vi "test_sound.vi"() -> ()   [LabVIEW 2019]
panel:
  in  "stop":bool
  out "frequency":dbl
  out "touch":dbl
  in  "stop (F)":bool
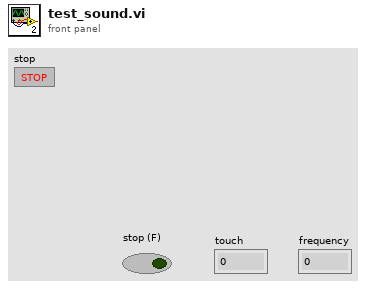
[diagram p1: front panel]
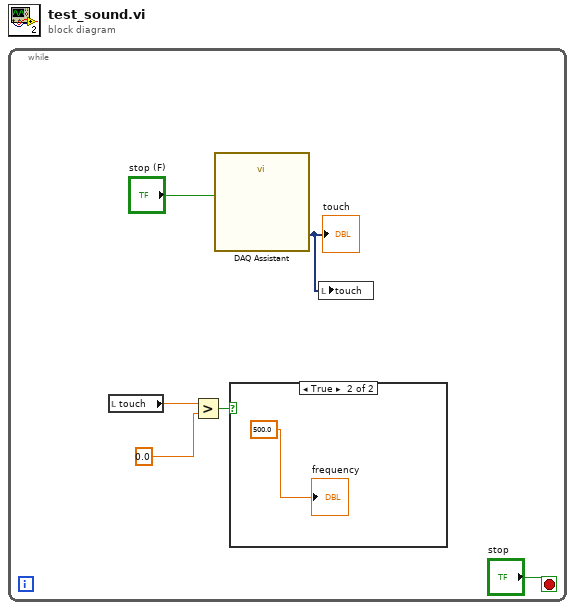
[diagram p0: block diagram]
diagram:
  n1 = while {
    stop <- "stop" stop-if-true
    n2 = local read "touch"() -> (w6:dbl)
    n3 = Greater?(x=w6, y=0.0) -> (0:w4:bool)
    n4 = call "DAQ Assistant"("stop (F)"="stop (F)") -> ("data"=w1:dynamicdata)  [unwired: 15 in, 3 out]
    "touch" <- w1
    n5 = case shown="True" w4 {
      frame False {
      }
      frame True {
        "frequency" <- 500.0 ("frequency")
      }
    }
    n6 = local write "touch"(w1) -> ()
  }
